vi "DB Tools Is DateTime String.vi"(3 "string or date/time":variant) -> (0 "database data type":T1, 1 "data":string)   [LabVIEW 2020, in "NI_Database_API.lvlib"]
doc: "Determines if a string is a timestamp. It checks for an initial sequence placed there by another subVI that formats timestamps. It returns the data type and the string."
uses:
  <vilib>/addons/database/NI_Database_API.lvlib
  <vilib>/addons/database/Auxilliary.llb/DB Tools DataTypes.ctl
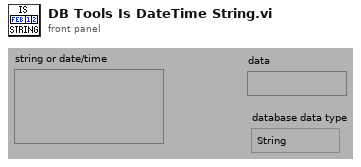
[diagram p1: front panel]
types:
  T1 = typedef "NI_Database_API.lvlib/DB Tools DataTypes.ctl" = enum16{"String", "Long (I32)", "Single (SGL)", "Double (DBL)", "Date/Time", "Binary"}
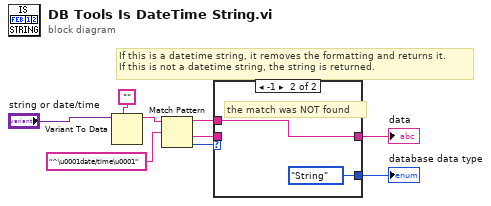
[diagram p0: block diagram]
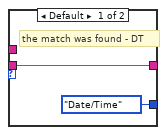
[diagram p2: hidden frame]
diagram:
  # "If this is a datetime string, it removes the formatting and returns it.  \nIf this is not a datetime string, the string is returned."
  n1 = Variant To Data(type="", Variant="string or date/time") -> (data=w7:string)  [unwired: 1 in, 1 out]
  n2 = Match Pattern(string=w7, regular expression="^\u0001date/time\u0001" ("string (\"\")")) -> (before substring=w4:string, after substring=w5:string, offset past match=w1:i32)  [unwired: 1 in, 1 out]
  n3 = case shown="-1" w1 {
    tunnel: w5 -> [w11 _]
    tunnel: w4 -> [_ w13]
    tunnel: [w11 w13] -> w3
    tunnel: [DB_Tools_DataTypes."Date/Time" ("database data type") DB_Tools_DataTypes."String" ("database data type")] -> w2
    frame Default {
      # "the match was found - DT"
    }
    frame -1 {
      # "the match was NOT found"
    }
  }
  "data" <- w3
  "database data type" <- w2
